vi "Ship Test Data Status.vi"(0 "Traceability 引用句柄":refnum<k24>, 1 "SeqNo":string, 2 "OperatorName":string, 5 "SNID":string, 7 "ItemID":string, 9 "Process":string, 11 "error in (no error)":errorcluster caption="错误输入（无错误）", 12 "Path":string) -> (4 "Traceability 引用句柄输出":refnum<k24>, 6 "ShipTestDataStatus":string, 15 "error out":errorcluster caption="错误输出")   [LabVIEW 2014, in "Traceability.lvlib"]
uses:
  D:/webservice/Traceability.dll
  Traceability.dll
  Traceability.lvlib
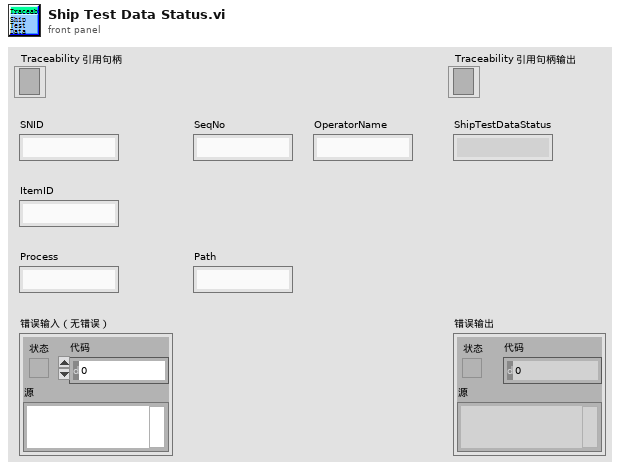
[diagram p1: front panel]
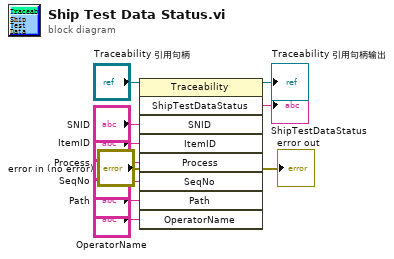
[diagram p0: block diagram]
diagram:
  n1 = invoke class="Traceability" method="ShipTestDataStatus"(reference="Traceability 引用句柄", error in="error in (no error)", "SNID"="SNID", "ItemID"="ItemID", "Process"="Process", "SeqNo"="SeqNo", "Path"="Path", "OperatorName"="OperatorName") -> (reference out=→"Traceability 引用句柄输出":refnum<k24>, error out=→"error out":errorcluster, "ShipTestDataStatus"=→"ShipTestDataStatus":string)  [unwired: 1 in, 6 out]
